vi "kvCanWrite.vi"(0 "Channel Handle (input only)":i32, 1 "Message Id":i32, 2 "Message":u8[](array[numeric]), 3 "DLC":u8, 5 "error in (no error)":errorcluster, 6 "Remote Request":bool, 7 "FD Frame":bool, 8 "Standard 11-bit Id":bool, 9 "Bit Rate Switch":bool, 10 "Extended 29-bit Id":bool, 11 "Single Shot":bool, 12 "Wakeup":bool, 13 "Error Frame":bool) -> (14 "Channel Handle (output only)":i32, 19 "error out":errorcluster)   [LabVIEW 2022 SP3]
doc: "This function sends a CAN message. The call returns immediately after queuing the message to the driver.\n\nThe message has been queued for transmission when this calls return. It has not necessarily been sent."
uses:
  canlib32.dll
panel:
  # "Set zero or more message flags."
  # "8"
  # "16"
  # "24"
  # "32"
  # "40"
  # "48"
  # "56"
  # "64"
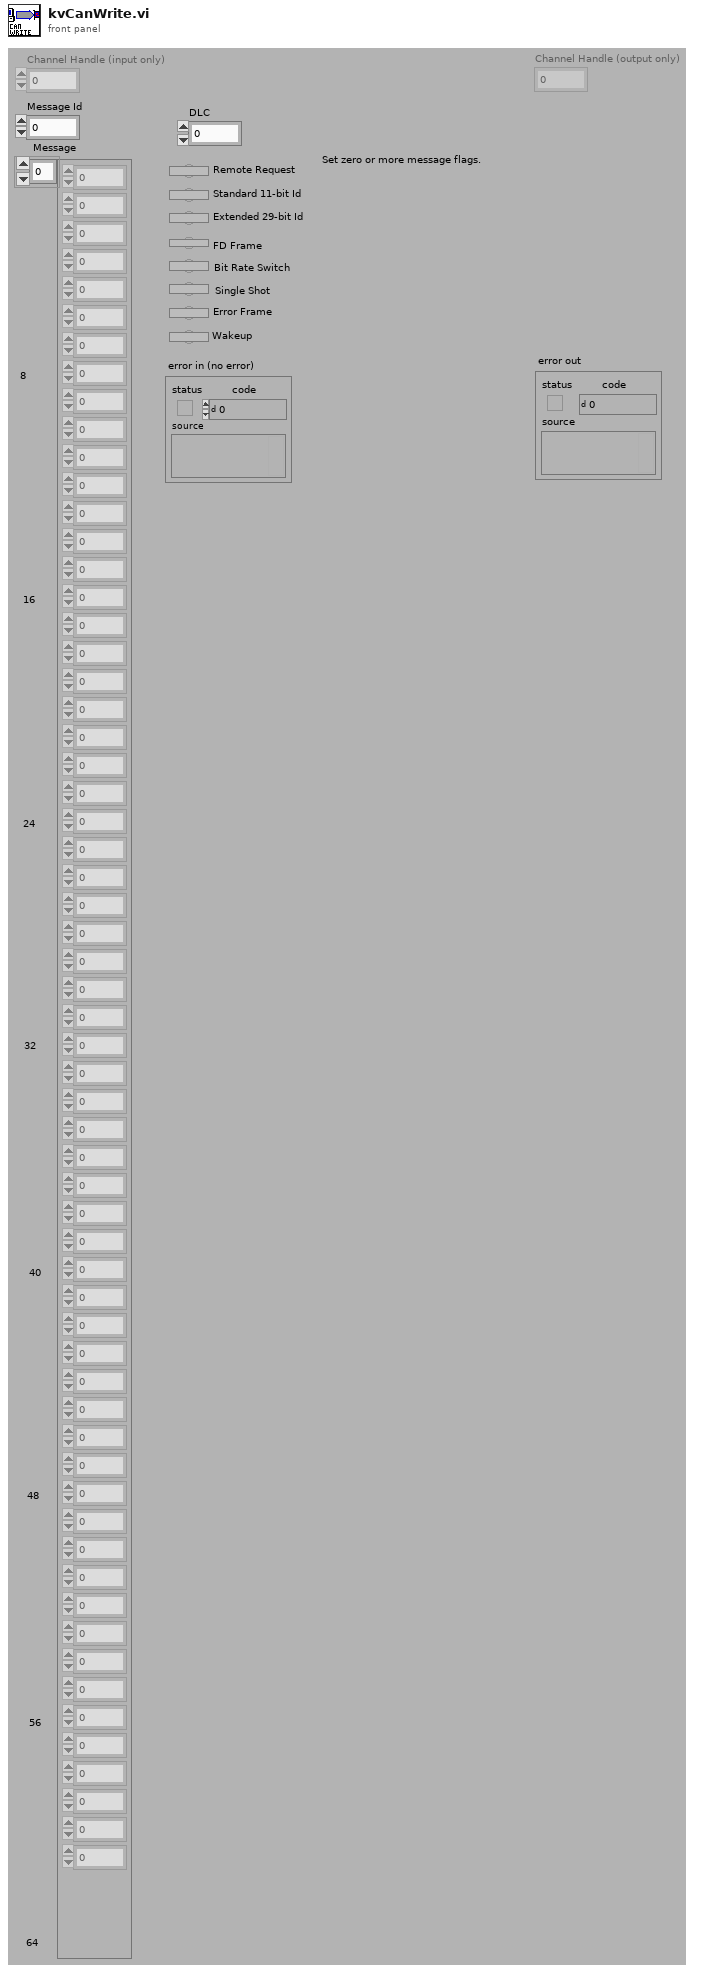
[diagram p1: front panel]
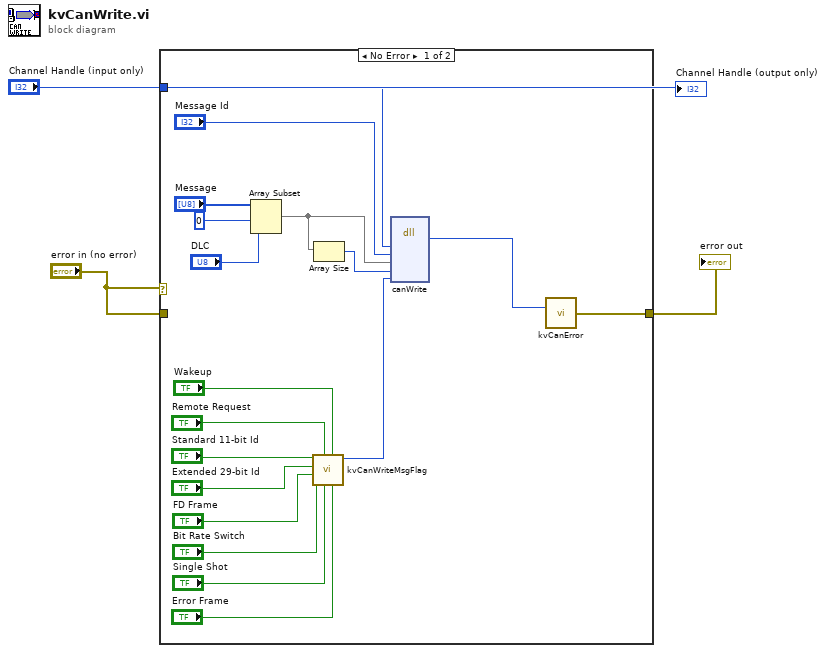
[diagram p0: block diagram]
diagram:
  n1 = case shown="No Error" "error in (no error)" {
    tunnel: [w11 w22] -> w2
    tunnel: "error in (no error)" -> [_ w22]
    tunnel: "Channel Handle (input only)" -> [w9 _]
    frame No Error {
      n2 = Array Subset(array="Message", index=0, length="DLC") -> (w14:u8[])
      n3 = call "kvCanWriteMsgFlag.vi"("Error Frame"="Error Frame", "Wakeup"="Wakeup", "Single Shot"="Single Shot", "Remote Request"="Remote Request", "Bit Rate Switch"="Bit Rate Switch", "FD Frame"="FD Frame", "Extended 29-bit Id"="Extended 29-bit Id", "Standard 11-bit Id"="Standard 11-bit Id") -> ("Flag Value"=w12:u32)  [unwired: 3 in]
      n4 = Array Size(array=w14) -> (size(s)=w13:i32)
      n5 = dll-call lib="canlib32.dll" fn="canWrite"("handle"=w9, "id"="Message Id", "msg"=w14, "dlc"=w13, "flag"=w12) -> (w10:i32)  [unwired: 8 in, 2 out]
      n6 = call "kvCanError.vi"("error code"=w10) -> ("error out"=w11:errorcluster)
    }
    frame Error {
    }
  }
  "error out" <- w2
  "Channel Handle (output only)" <- "Channel Handle (input only)"
